vi "set file meta.vi"(8 "error in (no error)":errorcluster, 11 "USRP_1_x_200MHz in":refnum<class "USRP_1_x_200MHz.lvclass">) -> (0 "error out":errorcluster, 3 "USRP_1_x_200MHz out":refnum<class "USRP_1_x_200MHz.lvclass">)   [LabVIEW 2021, in "USRP_1_x_200MHz.lvclass"]
uses:
  USRP_1_x_200MHz.lvclass
  USRP_1_x_200MHz.lvclass/USRP_1_x_200MHz.ctl
  pulse_tx_vis/device_mode.ctl
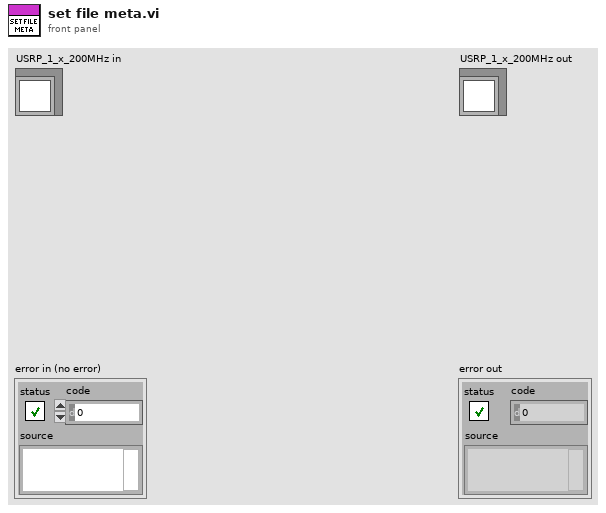
[diagram p1: front panel]
types:
  T1 = typedef "device_mode.ctl" = enum16{"USRP - 180MHz", "5785 - 2*180MHz", "5785 - 3.2GHz", "P2P - VST"}
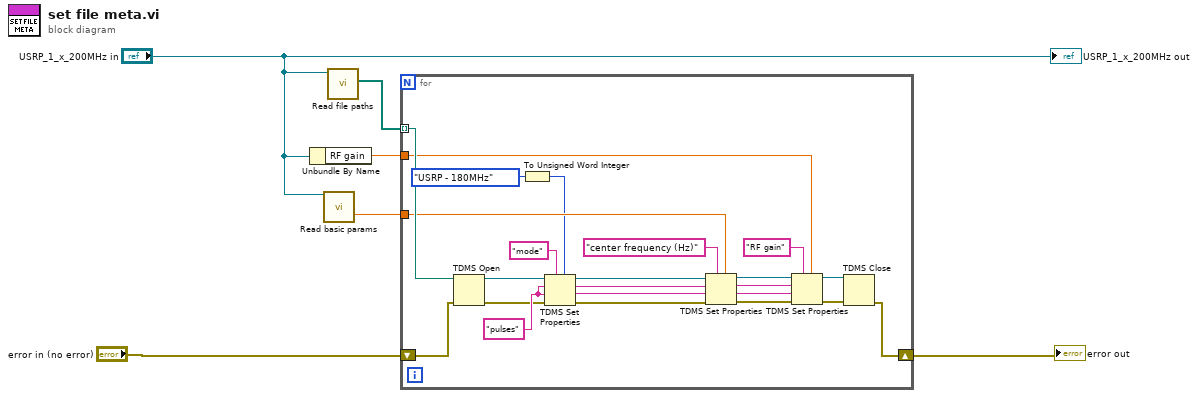
[diagram p0: block diagram]
diagram:
  n1 = Unbundle By Name("USRP_1_x_200MHz in") -> ("RF gain"=w1:dbl)
  n2 = call-dynamic "Read basic params.vi"("device_type in"="USRP_1_x_200MHz in") -> ("center frequency (Hz)"=w5:dbl)  [unwired: 13 in, 5 out]
  n3 = call-dynamic "Read file paths.vi"("device_type in"="USRP_1_x_200MHz in") -> ("file paths"=w6:path[])  [unwired: 8 in, 2 out]
  n4 = for {
    tunnel: w6 -> [w27] mode=indexing
    shift-right: [w17] -> w3
    shift-left: "error in (no error)" -> [w18]
    tunnel: w5 -> [w19]
    tunnel: w1 -> [w13]
    w29 = "pulses" ("channel name")
    n5 = TDMS Open(8:w18, 11:w27) -> (0:w26:errorcluster, 3:w28:refnum<k34>)  [unwired: 5 in]
    n6 = To Unsigned Word Integer(number=device_mode."USRP - 180MHz" ("Mode")) -> (unsigned 16bit integer=w7:u16)
    n7 = TDMS Set Properties(5:w7, 7:"mode", 8:w26, 9:w29, 10:w29, 11:w28) -> (0:w23:errorcluster, 1:w22:string, 2:w21:string, 3:w24:refnum<k34>)
    n8 = TDMS Set Properties(5:w19, 7:"center frequency (Hz)", 8:w23, 9:w22, 10:w21, 11:w24) -> (0:w9:errorcluster, 1:w10:string, 2:w11:string, 3:w12:refnum<k34>)
    n9 = TDMS Set Properties(5:w13, 7:"RF gain", 8:w9, 9:w10, 10:w11, 11:w12) -> (0:w15:errorcluster, 3:w14:refnum<k34>)  [unwired: 2 out]
    n10 = TDMS Close(8:w15, 11:w14) -> (0:w17:errorcluster)  [unwired: 1 out]
  }
  "error out" <- w3
  "USRP_1_x_200MHz out" <- "USRP_1_x_200MHz in"
